vi "main.vi"(8 "error in":errorcluster) -> (0 "error out":errorcluster)   [LabVIEW 2018, in "template.lvlib"]
uses:
  template.lvlib
  Common/Common.lvlib
  Common/vi/Stop All - Action.ctl
  ctl/Queue Actions.ctl
  ctl/Module State.ctl
  Error Handler/Error Handler/ctl/Module State.ctl
  Error Handler/Error Handler/Error Handler.lvlib
  Controller/Controller.lvlib
  Controller/ctl/Module State.ctl
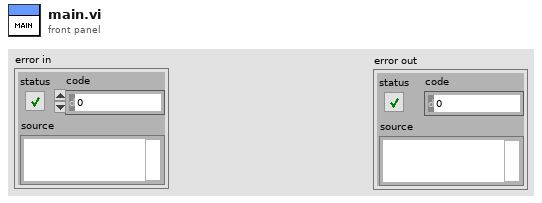
[diagram p1: front panel]
types:
  T1 = typedef "template.lvlib/Module State.ctl" = enum16{"Init", "Idle", "Error", "Close"}
  T2 = typedef "template.lvlib/Queue Actions.ctl" = enum16{"Create", "Get", "Destroy"}
  T3 = typedef "Common.lvlib/Stop All - Action.ctl" = enum16{"Create", "Get", "Fire", "Destroy"}
  T4 = typedef "Controller.lvlib/Module State.ctl" = enum16{"Init", "Idle", "Error", "Close"}
  T5 = typedef "Error Handler.lvlib/Module State.ctl" = enum16{"Init", "Idle", "Error", "Close", "Handle External Error", "Log Error"}
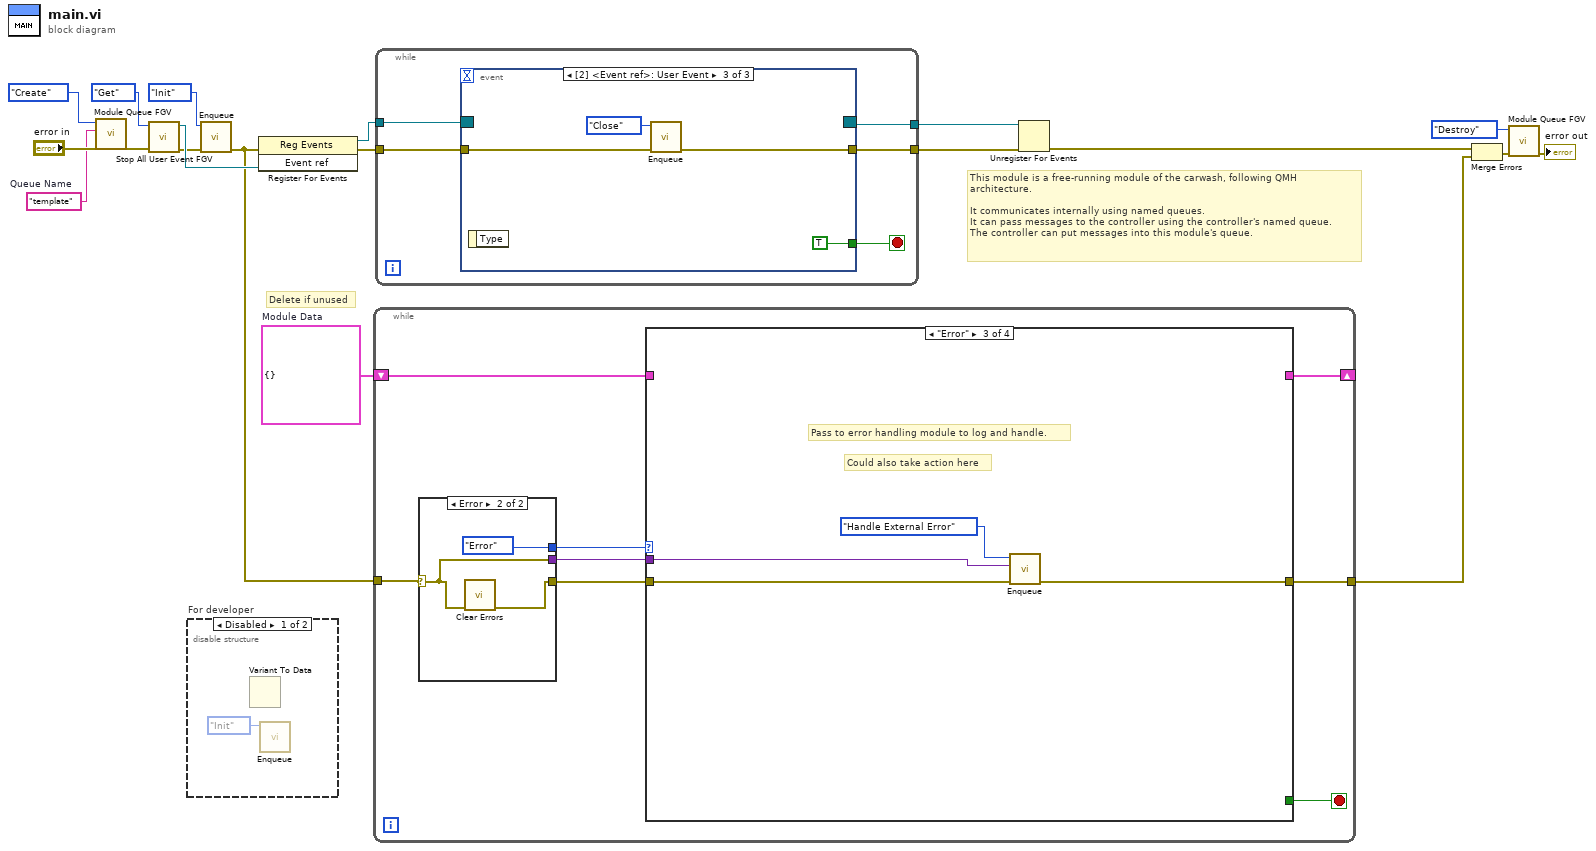
[diagram p0: block diagram]
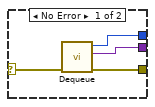
[diagram p3: hidden frame]
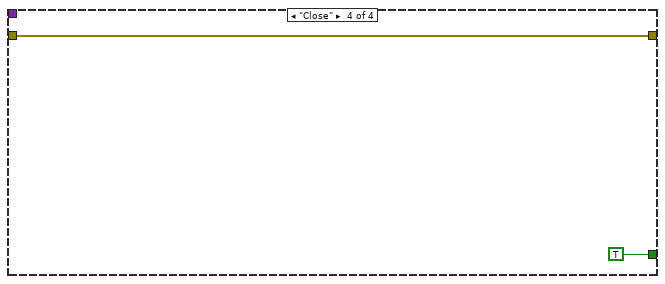
[diagram p6: hidden frame]
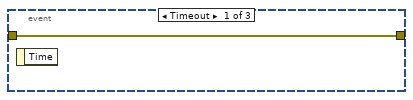
[diagram p7: hidden frame]
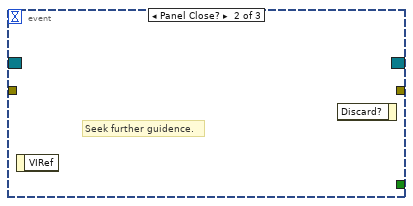
[diagram p8: hidden frame]
diagram:
  w1 = "template"  # Queue Name
  w6 = cluster{} {}  # Module Data
  # "This module is a free-running module of the carwash, following QMH\narchitecture.\n\nIt communicates internally using named queues.\nIt can pass messages to the controller using the controller's named queue.\nThe controller can put messages into this module's queue."
  # "Delete if unused"
  n1 = call "Module Queue FGV.vi"("error in"="error in", "Queue Name"=w1, "Action"=Queue_Actions."Create") -> ("error out"=w16:errorcluster)  [unwired: 7 in, 1 out]
  n2 = call "Stop All User Event FGV.vi"("error in"=w16, "Action"=Stop_All_-_Action."Get") -> ("error out"=w15:errorcluster, "Event ref"=w18:refnum<user-event>)  [unwired: 8 in]
  n3 = disable-structure "For developer" shown="Disabled" {
    frame Disabled {
      n4 = Variant To Data() -> ()  [unwired: 3 in, 2 out]
      n5 = call "Enqueue.vi"("State"=Module_State."Init") -> ()  [unwired: 10 in, 1 out]
    }
    frame Enabled {
    }
  }
  n6 = call "Enqueue.vi"("error in"=w15, "State"=Module_State."Init") -> ("error out"=w7:errorcluster)  [unwired: 9 in]
  n7 = register-events(error in=w7, w18) -> (reference out=w13:refnum<event-registration>, error out=w11:errorcluster)  [unwired: 1 in]
  n8 = while {
    tunnel: w7 -> [w28]
    shift-right: [w23] -> _
    shift-left: w6 -> [w24]
    tunnel: [w21] -> w5
    stop <- w22 stop-if-true
    n9 = case shown="Error" w28 {
      selector: w28 -> [w32 w33]
      tunnel: [w31 w34] -> w25
      tunnel: [w30 w33] -> w26
      tunnel: [w29 Module_State."Error" ("State")] -> w27
      frame No Error {
        n10 = call "Dequeue.vi"("error in"=w32) -> ("error out"=w31:errorcluster, "Data"=w30:variant, "State"=w29:T1)  [unwired: 8 in]
      }
      frame Error {
        n11 = call <vilib>:"Clear Errors.vi"("error in (no error)"=w33) -> ("error out"=w34:errorcluster)  [unwired: 5 in, 1 out]
      }
    }
    n12 = case shown="\"Error\"" w27 {
      tunnel: w26 -> [_ _ w38 _]
      tunnel: w25 -> [_ _ w37 w41]
      tunnel: w24 -> [_ w36 _ _]
      tunnel: [_ w36 _ _] -> w23
      tunnel: [_ _ _ TRUE] -> w22
      tunnel: [_ _ w39 w41] -> w21
      frame "Init", Default {
      }
      frame "Idle" {
      }
      frame "Error" {
        # "Could also take action here"
        # "Pass to error handling module to log and handle."
        n13 = call "Enqueue.vi"("error in"=w37, "Data"=w38, "State"=Module_State."Handle External Error") -> ("error out"=w39:errorcluster)  [unwired: 8 in]
      }
      frame "Close" {
      }
    }
  }
  n14 = while {
    tunnel: w13 -> [w47]
    tunnel: [w46] -> w12
    tunnel: [w45] -> w10
    tunnel: w11 -> [w44]
    stop <- w43 stop-if-true
    n15 = event shown="[2] <Event ref>: User Event" {
      selector: w47 -> [_ _ _]
      dyn-events: [_ _ _] -> w46
      timeout: _ -> [_ _ _]
      tunnel: [w48 _ w51] -> w45
      tunnel: w44 -> [w48 _ w52]
      tunnel: [_ _ TRUE] -> w43
      event Timeout {
        n16 = event-data() -> ()  [unwired: 1 in, 1 out]
      }
      event Panel Close? {
        # "Seek further guidence."
        n17 = event-data() -> ()  [unwired: 1 in, 1 out]
        n18 = event-data() -> ()  [unwired: 2 in, 1 out]
      }
      event User Event {
        n19 = event-data() -> ()  [unwired: 1 in, 1 out]
        n20 = call "Enqueue.vi"("error in"=w52, "State"=Module_State."Close") -> ("error out"=w51:errorcluster)  [unwired: 9 in]
      }
    }
  }
  n21 = Unregister For Events(event registration refnum=w12, error in=w10) -> (error out=w2:errorcluster)
  n22 = Merge Errors(w2, w5) -> (w4:errorcluster)
  n23 = call "Module Queue FGV.vi"("error in"=w4, "Action"=Queue_Actions."Destroy") -> ("error out"=→"error out":errorcluster)  [unwired: 8 in, 1 out]
